vi "Set All Plot Visibility (XYGraph).vi"(8 "error in (no error)":errorcluster, 10 "All Visible?":bool, 11 "XYGraph in":refnum<vi>) -> (0 "error out":errorcluster, 3 "XYGraph out":refnum<vi>)   [LabVIEW 2019, in "Instrument.Lockin.UI.lvclass"]
uses:
  Instrument.Lockin.UI.lvclass
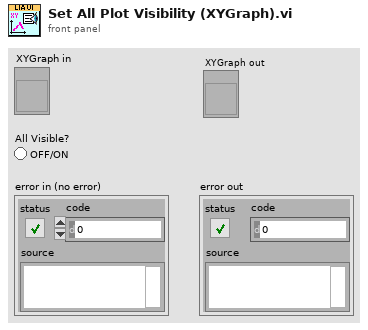
[diagram p1: front panel]
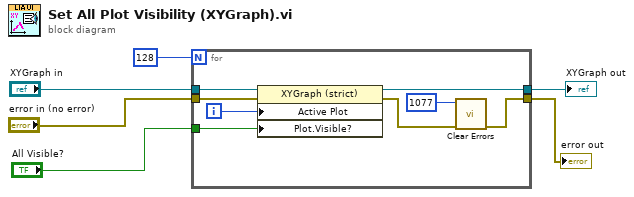
[diagram p0: block diagram]
diagram:
  n1 = for {
    N: 128 -> [_]
    tunnel: "XYGraph in" -> [w7]
    tunnel: [w13] -> w3
    tunnel: "error in (no error)" -> [w8]
    tunnel: [w12] -> w1
    tunnel: "All Visible?" -> [w9]
    i -> [w11]
    n2 = property on="Property Node" class="XYGraph (strict)"(reference=w7, error in=w8, "Active Plot"=w11, "Plot.Visible?"=w9) -> (reference out=w12:refnum<vi>, error out=w10:errorcluster)
    n3 = call <vilib>:"Clear Errors.vi"("error in (no error)"=w10, "specific error code to clear (0: all)"=1077) -> ("error out"=w13:errorcluster)  [unwired: 4 in, 1 out]
  }
  "error out" <- w3
  "XYGraph out" <- w1
